vi "LVIS_CheckResult.vi"(8 "Error In":errorcluster, 10 "CRC":string, 11 "Response":string) -> (0 "Error out":errorcluster, 1 "Online?":bool, 2 "SAF State":T1=99 items=["Clear"=0, "SAF Active"=100, "SAF Complete"=101, "SAF > 50%"=102, "SAF < 50%"=103, "SAF Full"=104, "Unknown"=99], 3 "Success?":bool)   [LabVIEW 2015]
doc: "Checks the Data Commander response for issues or errors."
uses:
  Ctrls/LVIS_SAF Status.ctl
  Globals/LVIS_DcGlobals.vi
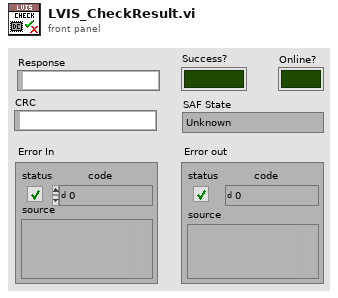
[diagram p1: front panel]
types:
  T1 = typedef "LVIS_SAF Status.ctl" = u16
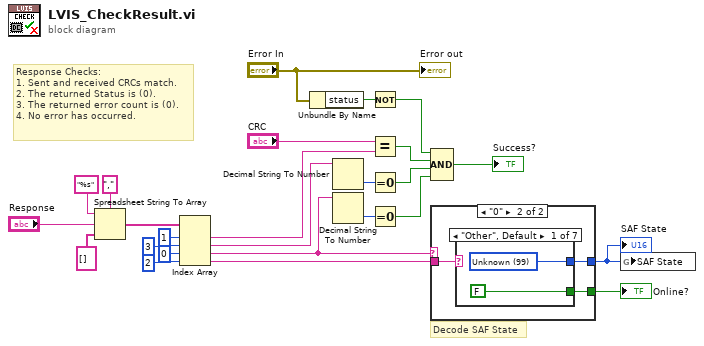
[diagram p0: block diagram]
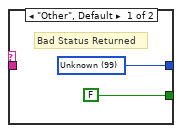
[diagram p2: hidden frame]
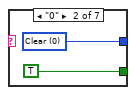
[diagram p3: hidden frame]
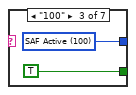
[diagram p4: hidden frame]
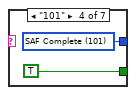
[diagram p5: hidden frame]
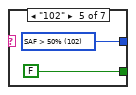
[diagram p6: hidden frame]
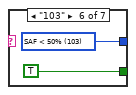
[diagram p7: hidden frame]
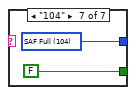
[diagram p8: hidden frame]
diagram:
  # "Decode SAF State"
  # "Response Checks:\n1. Sent and received CRCs match.\n2. The returned Status is (0).\n3. The returned error count is (0).\n4. No error has occurred."
  n1 = Spreadsheet String To Array(delimiter (Tab)=",", format string="%s", spreadsheet string="Response", array type (2D Dbl)=string[] []) -> (array=w22:string[])
  n2 = Index Array(array=w22, index #1=1 ("index"), index #2=3 ("index"), index #3=0 ("index"), index #4=2 ("index")) -> (element #1=w4:string, element #2=w3:string, element #3=w2:string, element #4=w9:string)
  n3 = Unbundle By Name("Error In") -> ("status"=w8:bool)
  n4 = Decimal String To Number(string=w3) -> (number=w20:i32)  [unwired: 2 in, 1 out]
  n5 = Decimal String To Number(string=w2) -> (number=w15:i32)  [unwired: 2 in, 1 out]
  n6 = Not(x=w8) -> (.not. x?=w7:bool)
  n7 = Equal?(x="CRC", y=w4) -> (x = y?=w14:bool)
  n8 = Equal To 0?(x=w20) -> (x = 0?=w13:bool)
  n9 = Equal To 0?(x=w15) -> (x = 0?=w12:bool)
  n10 = Compound Arithmetic op=AND(w7, w14, w13, w12) -> (→"Success?":bool)
  n11 = case shown="\"0\"" w2 {
    tunnel: w9 -> [_ w30]
    tunnel: [w27 w29] -> w11
    tunnel: [FALSE w28] -> w10
    frame "Other", Default {
      w27 = T1 99 items=["Clear"=0, "SAF Active"=100, "SAF Complete"=101, "SAF > 50%"=102, "SAF < 50%"=103, "SAF Full"=104, "Unknown"=99] ("SAF Status")
      # "Bad Status Returned"
    }
    frame "0" {
      n12 = case shown="\"Other\", Default" w30 {
        tunnel: [w32 w34 w36 w38 w40 w42 w44] -> w29
        tunnel: [FALSE TRUE TRUE TRUE FALSE TRUE FALSE] -> w28
        frame "Other", Default {
          w32 = T1 99 items=["Clear"=0, "SAF Active"=100, "SAF Complete"=101, "SAF > 50%"=102, "SAF < 50%"=103, "SAF Full"=104, "Unknown"=99] ("SAF Status")
        }
        frame "0" {
          w34 = T1 0 items=["Clear"=0, "SAF Active"=100, "SAF Complete"=101, "SAF > 50%"=102, "SAF < 50%"=103, "SAF Full"=104, "Unknown"=99] ("SAF Status")
        }
        frame "100" {
          w36 = T1 100 items=["Clear"=0, "SAF Active"=100, "SAF Complete"=101, "SAF > 50%"=102, "SAF < 50%"=103, "SAF Full"=104, "Unknown"=99] ("SAF Status")
        }
        frame "101" {
          w38 = T1 101 items=["Clear"=0, "SAF Active"=100, "SAF Complete"=101, "SAF > 50%"=102, "SAF < 50%"=103, "SAF Full"=104, "Unknown"=99] ("SAF Status")
        }
        frame "102" {
          w40 = T1 102 items=["Clear"=0, "SAF Active"=100, "SAF Complete"=101, "SAF > 50%"=102, "SAF < 50%"=103, "SAF Full"=104, "Unknown"=99] ("SAF Status")
        }
        frame "103" {
          w42 = T1 103 items=["Clear"=0, "SAF Active"=100, "SAF Complete"=101, "SAF > 50%"=102, "SAF < 50%"=103, "SAF Full"=104, "Unknown"=99] ("SAF Status")
        }
        frame "104" {
          w44 = T1 104 items=["Clear"=0, "SAF Active"=100, "SAF Complete"=101, "SAF > 50%"=102, "SAF < 50%"=103, "SAF Full"=104, "Unknown"=99] ("SAF Status")
        }
      }
    }
  }
  "SAF State" <- w11
  "Online?" <- w10
  n13 = global write "LVIS_DcGlobals.vi" "SAF State"(w11) -> ()
  "Error out" <- "Error In"
